vi "Get LakeShore 340 Manual.vi"(8 "error in (no error)":errorcluster, 10 "Output #":i32=1, 11 "VISA Resource Name":refnum<visa-resource-name>) -> (0 "error out":errorcluster, 2 "Manual otput":dbl, 3 "VISA Resource Name Out":refnum<visa-resource-name>)   [LabVIEW 2021]
uses:
  GPIB/VISA  Send Receive.vi
  Simple VISA Reader/Simple VISA Reader Driver.lvclass
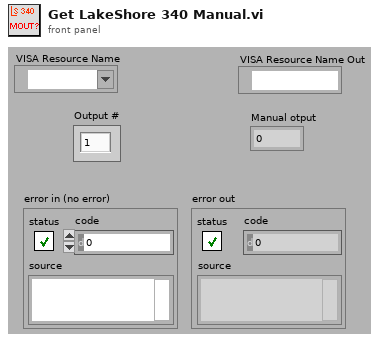
[diagram p1: front panel]
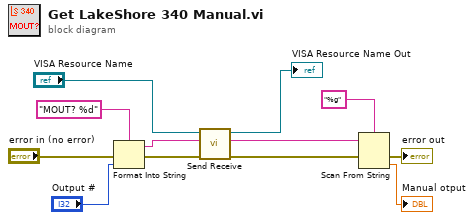
[diagram p0: block diagram]
diagram:
  n1 = Format Into String(format string="MOUT? %d" ("data string"), error in="error in (no error)", "Output #") -> (resulting string=w6:string, error out=w9:errorcluster)  [unwired: 1 in]
  n2 = call-poly "Send Receive.vi"("error in (no error)"=w9, "data string in"=w6, "VISA Resource Name"="VISA Resource Name") -> ("error out"=w4:errorcluster, "data string out"=w1:string, "VISA Resource Name Out"=→"VISA Resource Name Out":refnum<visa-resource-name>)  [unwired: 6 in]
  n3 = Scan From String(format string="%g", input string=w1, error in=w4) -> (error out=→"error out":errorcluster, output 1=→"Manual otput":dbl)  [unwired: 2 in, 2 out]
